vi "Trigger gRPC Connect Event.vi"(8 "error in (no error)":errorcluster, 10 "gRPC Connection Data":T1, 11 "CIF_Manager_UI in":refnum<class "CIF_Manager_UI.lvclass">) -> (0 "error out":errorcluster)   [LabVIEW 2021, in "CIF_Manager_UI.lvclass"]
uses:
  CIF_Manager_UI.lvclass
  <vilib>/gRPC/LabVIEW gRPC Library/Shared/grpcId.ctl
  <vilib>/gRPC/LabVIEW gRPC Library/grpc-lvsupport-release.lvlib
  <vilib>/CIF Foundation/CIF Core/CIFUI/Typedef/New Connection Event Data.ctl
  <vilib>/CIF Foundation/CIF Core/CIFUI/CIF_UI.lvclass
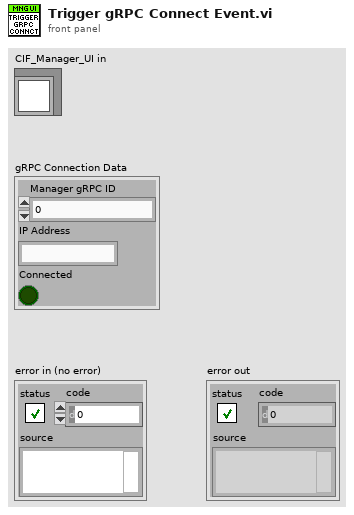
[diagram p1: front panel]
types:
  T1 = typedef "CIF_UI.lvclass/New Connection Event Data.ctl" = cluster{"Manager gRPC ID":T2, "IP Address":string, "Connected":bool}
  T2 = typedef "grpc-lvsupport-release.lvlib/grpcId.ctl" = u64
  T3 = typedef "CIF_UI.lvclass/SubPanel Events.ctl" = cluster{"Clear Local Error":refnum<user-event>, "Shutdown":refnum<user-event>, "gRPC Connection":refnum<user-event>, "Plugin Connection":refnum<user-event>}
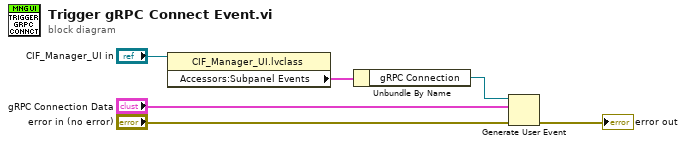
[diagram p0: block diagram]
diagram:
  n1 = property class="CIF_Manager_UI.lvclass"(reference="CIF_Manager_UI in") -> ("Accessors:Subpanel Events"=w4:T3)  [unwired: 1 in, 2 out]
  n2 = Unbundle By Name(w4) -> ("gRPC Connection"=w3:refnum<user-event>)
  n3 = Generate User Event(user event=w3, event data cluster="gRPC Connection Data", error in="error in (no error)") -> (error out=→"error out":errorcluster)  [unwired: 1 in, 1 out]
